vi "Set Data Name__ogtk.vi"(8 "error in (no error)":errorcluster, 9 "Data Name":string, 10 "Data":variant) -> (0 "error out":errorcluster, 2 "Renamed Data":variant)   [LabVIEW 2011]
doc: "Changes the data name of variant data."
panel:
  # "[OpenG VI Tags] ***Do Not Remove***"
  # "Set Data Name.vi\n\nChanges the data name of variant data.\n\nPlease visit http://www.OpenG.org to learn about the\nOpen Source LabVIEW software movement.\n\nNOTICE -- YOU MUST LEAVE THIS NOTICE IN PLACE.  PER THE TERMS OF THE LICENSE BELOW, YOU MAY SUBLICENSE THIS SOFTWARE \nIN ANY WAY THAT DOES NOT CONFLICT WITH THIS LICENSE.\n\n### BSD License (http://www.opensource.org/licenses/bsd-license.php) Begin ###\n \nCopyright (c) 2002, Jean-Pierre Drolet <drolet_jp@hotmail.com>\nCopyright (c) 2002-2006, Jim Kring <jim@jimkring.com>\n\nAll rights reserved.\n\nRedistribution and use in source and binary forms, with or without modification, are permitted provided that the following conditions are met:\n\n    * Redistributions of source code must retain the above copyright notice, this list of conditions and the following disclaimer.\n    * Redistributions in binary form must reproduce the above copyright notice, this list of conditions and the following disclaimer in the \n       documentation and/or other materials provided with the distribution.\n    * Neither the name of SciWare, James Kring, Inc., nor the names of its contributors may be used to endorse or promote products derived \n       from this software without specific prior written permission.\n\nTHIS SOFTWARE IS PROVIDED BY THE COPYRIGHT HOLDERS AND CONTRIBUTORS \"AS IS\" AND ANY EXPRESS OR IMPLIED WARRANTIES, \nINCLUDING, BUT NOT LIMITED TO, THE IMPLIED WARRANTIES OF MERCHANTABILITY AND FITNESS FOR A PARTICULAR PURPOSE ARE \nDISCLAIMED. IN NO EVENT SHALL THE COPYRIGHT OWNER OR CONTRIBUTORS BE LIABLE FOR ANY DIRECT, INDIRECT, INCIDENTAL,\n SPECIAL, EXEMPLARY, OR CONSEQUENTIAL DAMAGES (INCLUDING, BUT NOT LIMITED TO, PROCUREMENT OF SUBSTITUTE GOODS OR \nSERVICES; LOSS OF USE, DATA, OR PROFITS; OR BUSINESS INTERRUPTION) HOWEVER CAUSED AND ON ANY THEORY OF LIABILITY, \nWHETHER IN CONTRACT, STRICT LIABILITY, OR TORT (INCLUDING NEGLIGENCE OR OTHERWISE) ARISING IN ANY WAY OUT OF THE USE \nOF THIS SOFTWARE, EVEN IF ADVISED OF THE POSSIBILITY OF SUCH DAMAGE.\n\n### BSD License End ###"
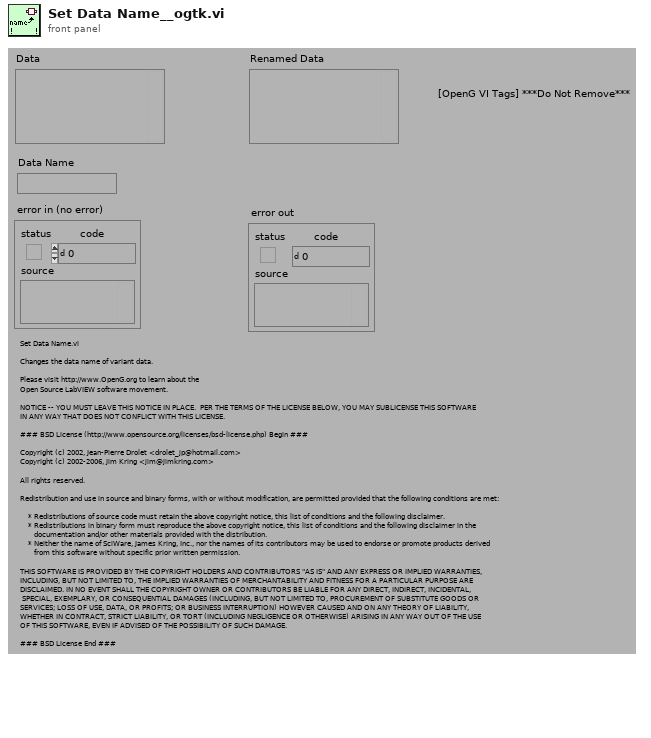
[diagram p1: front panel]
types:
  T1 = typedef "Type Descriptor Header__ogtk.ctl" = cluster{"length":u16, "private":u8, "type":T2, "# elements":u16}
  T2 = typedef "Type Descriptor Enumeration__ogtk.ctl" = enum8{"<Null>", "I8", "I16", "I32", "I64", "U8", "U16", "U32", "U64", "SGL", "DBL", "EXT", "CSG", "CDB", "CXT", "0x0F", "0x10", "0x11", "0x12", "0x13", "0x14", "Enum U8", "Enum U16", "Enum U32", "Enum U64", "SGL PQ", "DBL PQ", "EXT PQ", "CSG PQ", "CDB PQ", "CXT PQ", "0x1F", "0x20", "Boolean", "0x22", "0x23", "0x24", "0x25", "0x26", "0x27", "0x28", "0x29", "0x2A", "0x2B", "0x2C", "0x2D", "0x2E", "0x2F", "String", "0x31", "Path", "Pict", "0x34", "0x35", "0x36", "DAQ", "0x38", "0x39", "0x3A", "0x3B", "0x3C", "0x3D", "0x3E", "0x3F", "Array", "0x41", "0x42", "0x43", "0x44", "0x45", "0x46", "0x47", "0x48", "0x49", "0x4A", "0x4B", "0x4C", "0x4D", "0x4E", "0x4F", "Cluster", "0x51", "0x52", "Variant", "Waveform", "0x55", "0x56", "0x57", "0x58", "0x59", "0x5A", "0x5B", "0x5C", "0x5D", "0x5E", "0x5F", "0x60", "0x61", "0x62", "0x63", "0x64", "0x65", "0x66", "0x67", "0x68", "0x69", "0x6A", "0x6B", "0x6C", "0x6D", "0x6E", "0x6F", "Refnum"}
  T3 = typedef "Type Descriptor__ogtk.ctl" = i16[]
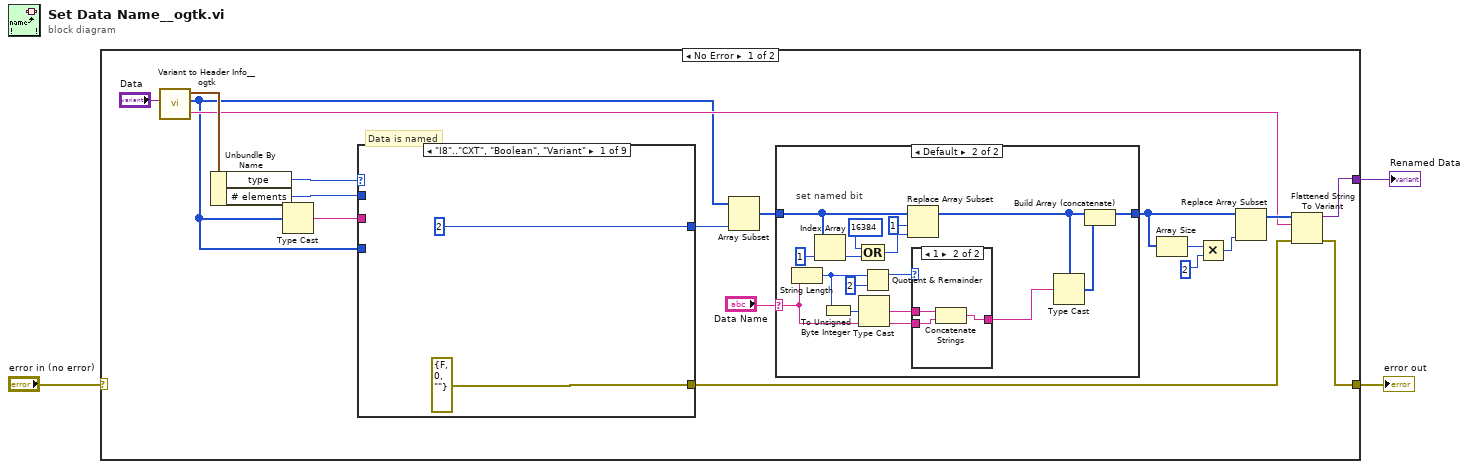
[diagram p0: block diagram]
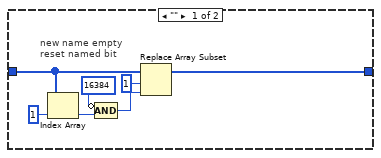
[diagram p2: hidden frame]
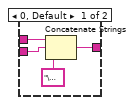
[diagram p3: hidden frame]
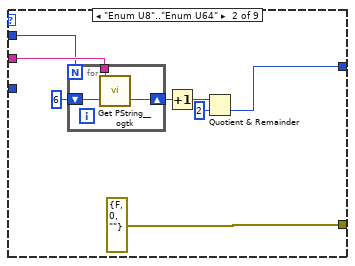
[diagram p4: hidden frame]
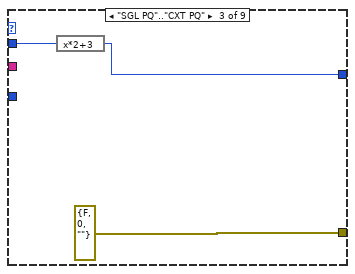
[diagram p5: hidden frame]
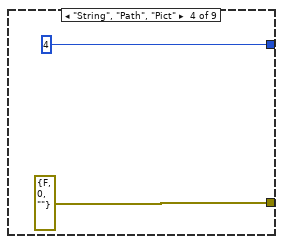
[diagram p6: hidden frame]
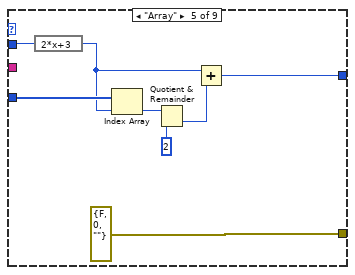
[diagram p7: hidden frame]
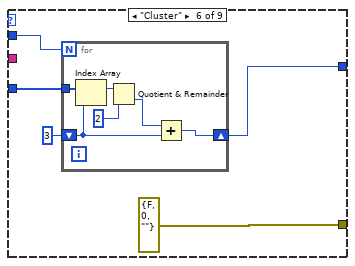
[diagram p8: hidden frame]
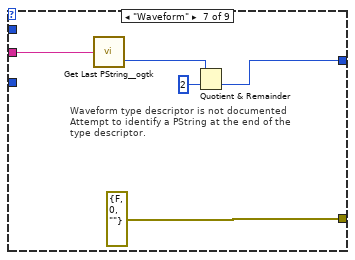
[diagram p9: hidden frame]
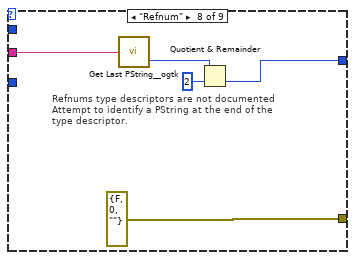
[diagram p10: hidden frame]
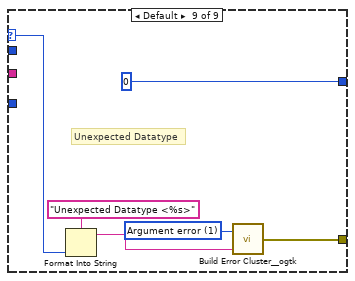
[diagram p11: hidden frame]
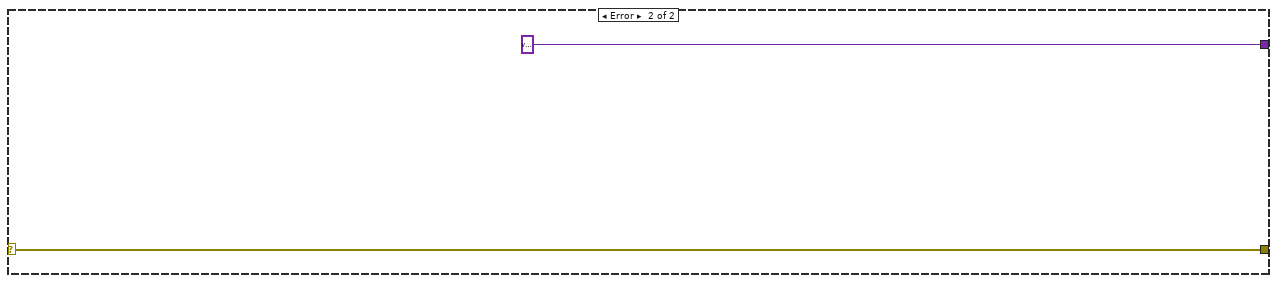
[diagram p12: hidden frame]
diagram:
  n1 = case shown="No Error" "error in (no error)" {
    selector: "error in (no error)" -> [_ w106]
    tunnel: [w6 w106] -> w3
    tunnel: [w8 variant ("Renamed Data")] -> w1
    frame No Error {
      # "Data is named"
      n2 = call "Variant to Header Info__ogtk.vi"("Variant"="Data") -> ("Type Descriptor Header"=w21:T1, "Type Descriptor"=w4:T3, "data string"=w7:string)  [unwired: 3 in]
      n3 = Unbundle By Name(w21) -> ("type"=w20:T2, "# elements"=w17:u16)
      n4 = Type Cast(x=w4) -> (*(type *) &x=w18:string)  [unwired: 1 in]
      n5 = case shown="\"I8\"..\"CXT\", \"Boolean\", \"Variant\"" w20 {
        selector: w20 -> [_ _ _ _ _ _ _ _ w101]
        tunnel: [errorcluster {"status"=FALSE, "code"=0, "source"=""} ("error out") errorcluster {"status"=FALSE, "code"=0, "source"=""} ("error out") errorcluster {"status"=FALSE, "code"=0, "source"=""} ("error out") errorcluster {"status"=FALSE, "code"=0, "source"=""} ("error out") errorcluster {"status"=FALSE, "code"=0, "source"=""} ("error out") errorcluster {"status"=FALSE, "code"=0, "source"=""} ("error out") errorcluster {"status"=FALSE, "code"=0, "source"=""} ("error out") errorcluster {"status"=FALSE, "code"=0, "source"=""} ("error out") w104] -> w5
        tunnel: w18 -> [_ w59 _ _ _ _ w92 w98 _]
        tunnel: w17 -> [_ w57 w67 _ w76 w81 _ _ _]
        tunnel: w4 -> [_ _ _ _ w75 w80 _ _ _]
        tunnel: [2 ("offset (0)") w54 w65 4 ("offset (0)") w70 w78 w89 w94 0 ("PString Offset")] -> w16
        frame "I8".."CXT", "Boolean", "Variant" {
        }
        frame "Enum U8".."Enum U64" {
          n6 = for {
            N: w57 -> [_]
            tunnel: w59 -> [w62]
            shift-right: [w63] -> w60
            shift-left: 6 -> [w64]
            n7 = call "Get PString__ogtk.vi"("offset (0)"=w64, "String"=w62) -> ("offset past PString"=w63:i32)  [unwired: 1 out]
          }
          n8 = Increment(x=w60) -> (x+1=w55:i32)
          n9 = Quotient & Remainder(x=w55, y=2) -> (floor(x/y)=w54:i32)  [unwired: 1 out]
        }
        frame "SGL PQ".."CXT PQ" {
          n10 = expression code="x*2+3"(w67) -> (w65:u16)
        }
        frame "String", "Path", "Pict" {
        }
        frame "Array" {
          n11 = expression code="2*x+3"(w76) -> (w71:u16)
          n12 = Index Array(array=w75, index=w71) -> (element=w73:i16)
          n13 = Quotient & Remainder(x=w73, y=u16 2) -> (floor(x/y)=w72:u16)  [unwired: 1 out]
          n14 = Add(x=w71, y=w72) -> (x+y=w70:u16)
        }
        frame "Cluster" {
          n15 = for {
            N: w81 -> [_]
            shift-right: [w87] -> w78
            shift-left: i16 3 -> [w86]
            tunnel: w80 -> [w88]
            n16 = Index Array(array=w88, index=w86) -> (element=w84:i16)
            n17 = Quotient & Remainder(x=w84, y=i16 2) -> (floor(x/y)=w85:i16)  [unwired: 1 out]
            n18 = Add(x=w85, y=w86) -> (x+y=w87:i16)
          }
        }
        frame "Waveform" {
          # "Waveform type descriptor is not documented\nAttempt to identify a PString at the end of the\ntype descriptor."
          n19 = call "Get Last PString__ogtk.vi"("String"=w92) -> ("PString Offset"=w90:i32)  [unwired: 1 out]
          n20 = Quotient & Remainder(x=w90, y=2) -> (floor(x/y)=w89:i32)  [unwired: 1 out]
        }
        frame "Refnum" {
          # "Refnums type descriptors are not documented\nAttempt to identify a PString at the end of the\ntype descriptor."
          n21 = call "Get Last PString__ogtk.vi"("String"=w98) -> ("PString Offset"=w95:i32)  [unwired: 1 out]
          n22 = Quotient & Remainder(x=w95, y=2) -> (floor(x/y)=w94:i32)  [unwired: 1 out]
        }
        frame Default {
          w103 = 1 items=["No error", "Argument error", "Memory is full", "Out of zone", "End of file", "File already open", "Generic file I/O error", "File not found", "File permission error", "Disk is full", "Duplicate path", "Too many files open", "System feature not enabled", "Resource file not found", "Cannot add resource", "Resource not found", "Image not found", "Image memory error", "Pen does not exist", "Config type invalid", "Config token not found", "Config parse error", "Config memory error", "Bad external code format", "Bad external code offset", "External code not present", "Null window", "Destroy window error", "Null menu", "Print aborted", "Bad print record", "Print driver error", "Windows error during printing", "Memory error during printing", "Print dialog error", "Generic print error", "Invalid device refnum", "Device not found", "Device parameter error", "Device unit error", "Cannot open device", "Device call aborted", "Generic error", "Cancelled by user", "Object ID too low", "Object ID too high", "Object not in heap", "Unknown heap", "Unknown object (invalid DefProc)", "Unknown object (DefProc not in table)", "Message out of range", "Invalid (null) method", "Unknown message", "Manager call not supported", "Bad address", "Network operation in progress", "Network operation timed out", "Connection is busy", "Network attribute not supported", "Network error", "Address in use", "System out of memory", "Connection aborted", "Connection refused", "Not connected", "Already connected", "Connection closed", "Initialization error (interapplication manager)", "Bad occurrence", "Wait on unbound occurrence handler", "Occurrence queue overflow", "Datalog type conflict", "Unused", "Unrecognized type (interapplication manager)", "Memory corrupt", "Failed to make temporary DLL", "Old CIN version", "Drag socket not found", "Failed to load drop-object", "Failed to register OLE object", "Failed to release OLE object", "Format specifier type mismatch", "Unknown format specifier", "Too few format specifiers", "Too many format specifiers", "Scan failed", "Newer CIN version", "Error converting to variant", "Runtime menu error", "Password tampered", "Variant attribute not found", "Incompatible variant data type", "Event data is not available", "Event Store is not present", "Occurrence is not found", "Event Queue is not created", "Event info is not available", "Refnum passed is NULL", "Error retrieving Class GUID", "Error retrieving CoClass GUID", "Error retrieving TypeLib GUID.", "Bad built application magic bytes.", "Specific driver is different from the specific driver associated with the Logical Name.", "There is no session opened to the class driver.", "Max Error", "MAX - Error with config objects", "MAX - Error loading configuration", "MAX - Group not supported"]
          # "Unexpected Datatype"
          n23 = Format Into String(format string="Unexpected Datatype <%s>" ("Format String"), w101) -> (resulting string=w100:string)  [unwired: 2 in, 1 out]
          n24 = call "Build Error Cluster__ogtk.vi"("String to Prepend to source (\"\")"=w100, "code"=w103) -> ("error out"=w104:errorcluster)
        }
      }
      n25 = Array Subset(array=w4, length=w16) -> (w14:T3)  [unwired: 1 in]
      n26 = case shown="Default" "Data Name" {
        selector: "Data Name" -> [_ w36]
        tunnel: w14 -> [w28 w44]
        tunnel: [w23 w33] -> w10
        frame "" {
          # "new name empty\nreset named bit"
          n27 = Index Array(array=w28, index=1 ("Index")) -> (element=w26:i16)
          n28 = Compound Arithmetic op=AND(invert i16 16384 ("Input"), w26) -> (w25:i16)
          n29 = Replace Array Subset(array=w28, new element=w25, index=1 ("Index")) -> (w23:T3)
        }
        frame Default {
          # "set named bit"
          n30 = String Length(string=w36) -> (length=w32:i32)
          n31 = Index Array(array=w44, index=1 ("Index")) -> (element=w40:i16)
          n32 = To Unsigned Byte Integer(number=w32) -> (unsigned 8bit integer=w31:u8)
          n33 = Type Cast(x=w31) -> (*(type *) &x=w30:string)  [unwired: 1 in]
          n34 = Compound Arithmetic op=OR(i16 16384 ("Input"), w40) -> (w42:i16)
          n35 = Quotient & Remainder(x=w32, y=2) -> (x-y*floor(x/y)=w38:i32)  [unwired: 1 out]
          n36 = Replace Array Subset(array=w44, new element=w42, index=1 ("Index")) -> (w34:T3)
          n37 = case shown="1" w38 {
            tunnel: [w48 w49] -> w37
            tunnel: w36 -> [w47 w50]
            tunnel: w30 -> [w45 w51]
            frame 0, Default {
              n38 = Concatenate Strings(w45, w47, "\u0000" ("Substring")) -> (w48:string)
            }
            frame 1 {
              n39 = Concatenate Strings(w51, w50) -> (w49:string)
            }
          }
          n40 = Type Cast(type=w34, x=w37) -> (*(type *) &x=w35:T3)
          n41 = Build Array (concatenate)(w34, w35) -> (w33:T3)
        }
      }
      n42 = Array Size(array=w10) -> (size(s)=w13:i32)
      n43 = Multiply(x=w13, y=2) -> (x*y=w11:i32)
      n44 = Replace Array Subset(array=w10, new element=w11) -> (w9:T3)  [unwired: 1 in]
      n45 = Flattened String To Variant(4:w5, 6:w7, 7:w9) -> (0:w6:errorcluster, 3:w8:variant)
    }
    frame Error {
    }
  }
  "error out" <- w3
  "Renamed Data" <- w1
